vi "MASTER_QCM_O2_IM6_4200.vi"() -> ()   [LabVIEW 2013]
doc: "This example demonstrates temperature control and monitoring.\n\nNote:\nBefore start this VI is it necessary:\n\n- preconfigure some specific parameters that are not supported by this driver (e.g. PV-I/O Type, Linearization type, Alarm Input Values... ) by Quick Codes, or by Eurotherm iTools or by instrument front panel controls\n- enter correct VISA Resource Descriptor, Device Address and Baud Rate into front-panel controls"
uses:
  <vilib>/Instr/_visa.llb/VISA Event Mechanism.ctl
  <vilib>/Instr/_visa.llb/Select Event Type.ctl
  <vilib>/DAQmx/read.llb/DAQmx Read (Analog DBL 1Chan 1Samp).vi
  <vilib>/Utility/file.llb/Write To Spreadsheet File (string).vi
  LabVIEW Drivers for DVS instruments/Zahner VIs/IM/ZRemote-Globals.vi
  <vilib>/DAQmx/miscellaneous.llb/DAQmx Fill In Error Info.vi
panel:
  in  "Tab Control":T1(tab)
  in  "Add comments to the data file here and click anywhere outside the comment\nbox to save. The time at which the comment is saved is recorded in the data file.":string
  in  "O2 PUMP":bool
  in  "QCM":bool
  out "Program Errors":errorcluster
  out "Current Date/Time":string
  out "Starting Date/Time":string
  in  "Zahner IM6":bool
  in  "stop":bool
  in  "Quit VI":bool
  in  "Keithley 4200":bool
  out "Freq and Resistance Graph 2":T2(graph)
  out "Frequency (Hz)":dbl format="%.6e"
  out "Resistance (Ohm)":dbl format="%.6e"
  out "Waveform Chart 2":dbl(graph)
  out "Waveform Chart":cluster{dbl}(graph)
  out "Torr":dbl
  out "%":dbl
  out "atm":dbl
  out "O2 pump voltage":dbl format="%0.2f"
  in  "Com Port":i32(ring) items=["Com 1", "Com 2", "Com 3", "Com 4", "Com 5", "Com 6", "COM 7", "COM 8", "COM 9", "COM 10", "COM 11", "COM 12", "com 13", "COM 14"]
  in  "Baud Rate 2":i32(ring)=2 items=["2400", "4800", "9600", "19200", "38400", "57600", "115200"]
  out "Waveform Chart 3":cluster{dbl}(graph)
  out "XY Graph":cluster{dbl[], dbl[]}(graph)
  out "Current (A)    Voltage (V)":dbl[][](array[numeric]) caption="appended array"
  out "Resistance (Ohm)":dbl
  in  "Amplitude":dbl format="%.2p"
  in  "Period Count":i16=2 min=1 max=99
  in  "Frequency":dbl=1000.0 format="%.3p"
  out "Imaginary":dbl format="%.3p"
  out "Real":dbl format="%.3p"
  out "Potential Meter":dbl[unit](knob) scale=-10.0..10.0 scale format="%.0p"
  out "Current Meter":dbl[unit](knob) min=-2.0 max=2.0 step=1e-06 scale=-1e-06..1e-06 scale format="%.0p"
  in  "Measure OCP":bool
  in  "IP Address":string="127.0.0.1"
  in  "Device Name":string="ScriptRemote"
  in  "Galvanostat":bool
  in  "Set Current":dbl format="%.3p"
  in  "Potentiostat":bool=TRUE
  in  "Start IM remote":bool
  in  "Set Potential":dbl format="%.3p"
  in  "Device":i16 min=0 max=4
  in  "Measure EIS":bool
  in  "Cell Switch":bool
  in  "CV":bool
  in  "IE":bool
  in  "EIS":bool
  out "Busy":bool
  # "Configuring Instrument\n \nPlease Wait......\n\nChart will update in 20 sec"
  # "Instruments Connected"
  # "COMMENT BOX"
  # "Instructions:\n\nSelect the instruments above which are connected, turned on, and configured to record data.\n\nSet the file path destination for the data file produced by each instrument.\n\nRun the Pirani Control software, and make sure Pirani is saving a log of the temp/pressure/gas flow data. \n\nClick the RUN arrow on the LabVIEW toolbar, and wait for instruments to begin recording.\n\nTo end, click the red STOP button ONLY for instruments that are running.\n\nDO NOT press the STOP button on the toolbar."
  # "O2 Partial Pressure"
  # "V"
  # "4-Point Resistance Measurement:\nSMU1 = Current Source, Voltmeter\nSMU2 = COM & GND"
  # "Start Measurements"
  # "Impedance"
  # "Setup"
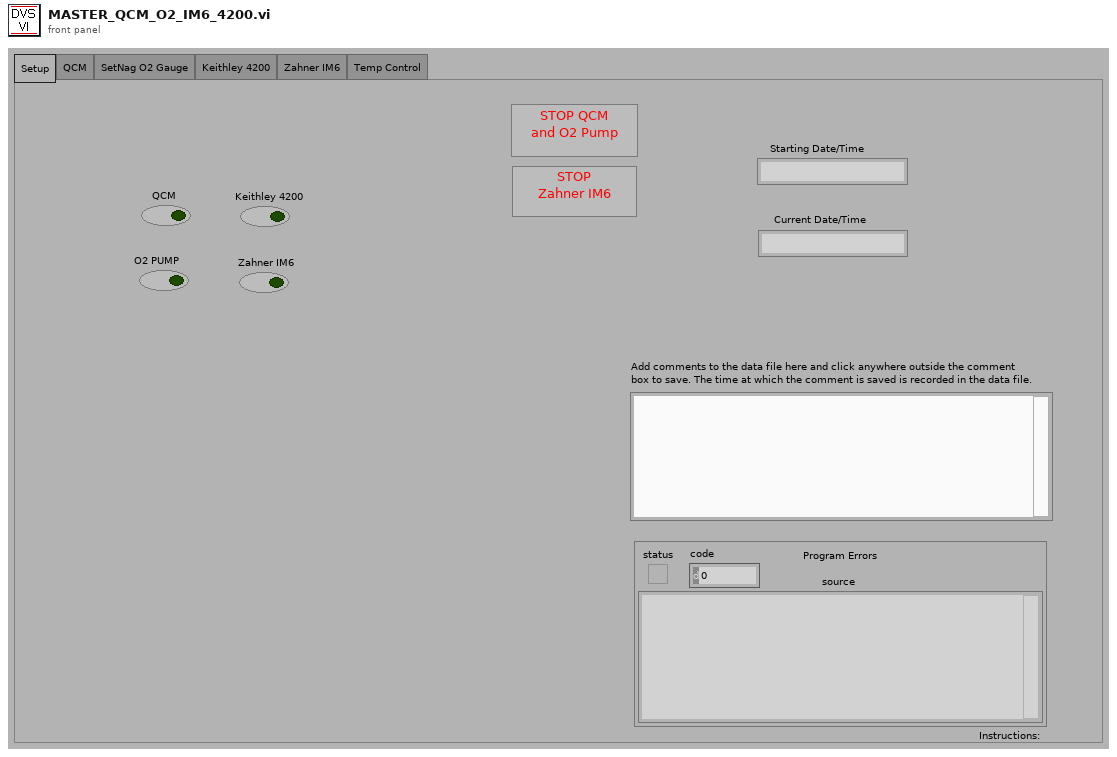
[diagram p1: front panel]
types:
  T1 = enum32{"Setup", "QCM", "SetNag O2 Gauge", "Keithley 4200", "Zahner IM6", "Temp Control"}
  T2 = cluster{"XY chart data":cluster{"x":dbl, "y":dbl}[]}[]
  T3 = enum16{"open", "open or create", "create or replace", "create", "open (read only)"}
  T4 = cluster{"IP Address":string, "Device Name":string, "Buffer Size":u16, "Start IM remote":bool}
  T5 = cluster{"Pset":dbl, "Cset":dbl, "Frq":dbl, "Ampl":dbl, "Nw":i16, "Pot":bool, "Gal":bool, "GAL":i16, "Cmin":dbl, "Cmax":dbl, "Pmin":dbl, "Pmax":dbl, "DEV":i16, "EPC":i16, "MAXDEV":i16}
  T6 = enum16{"no parity", "odd parity", "even parity", "mark parity", "space parity"}
  T7 = cluster{"Time Target (s)":dbl, "VISA in":refnum<visa-resource-name>, "error out":errorcluster}
  T8 = cluster{"Elapsed Time (s)":dbl, "VISA out":refnum<visa-resource-name>, "error out":errorcluster}
  T9 = typedef "Select Event Type.ctl" = u32
  T10 = typedef "VISA Event Mechanism.ctl" = u16
  T11 = cluster{"y":dbl, string, string, "error out":errorcluster}
  T12 = cluster{dbl, string, string, "error out":errorcluster}
  T13 = cluster{"error out":errorcluster, string, string}
  T14 = cluster{"timestamp out":dbl, "Frequency out":dbl}
  T15 = cluster{"timestamp out":dbl, "Resistance out":dbl}
  T16 = cluster{"error out":errorcluster, "error out":errorcluster, "error out":errorcluster}
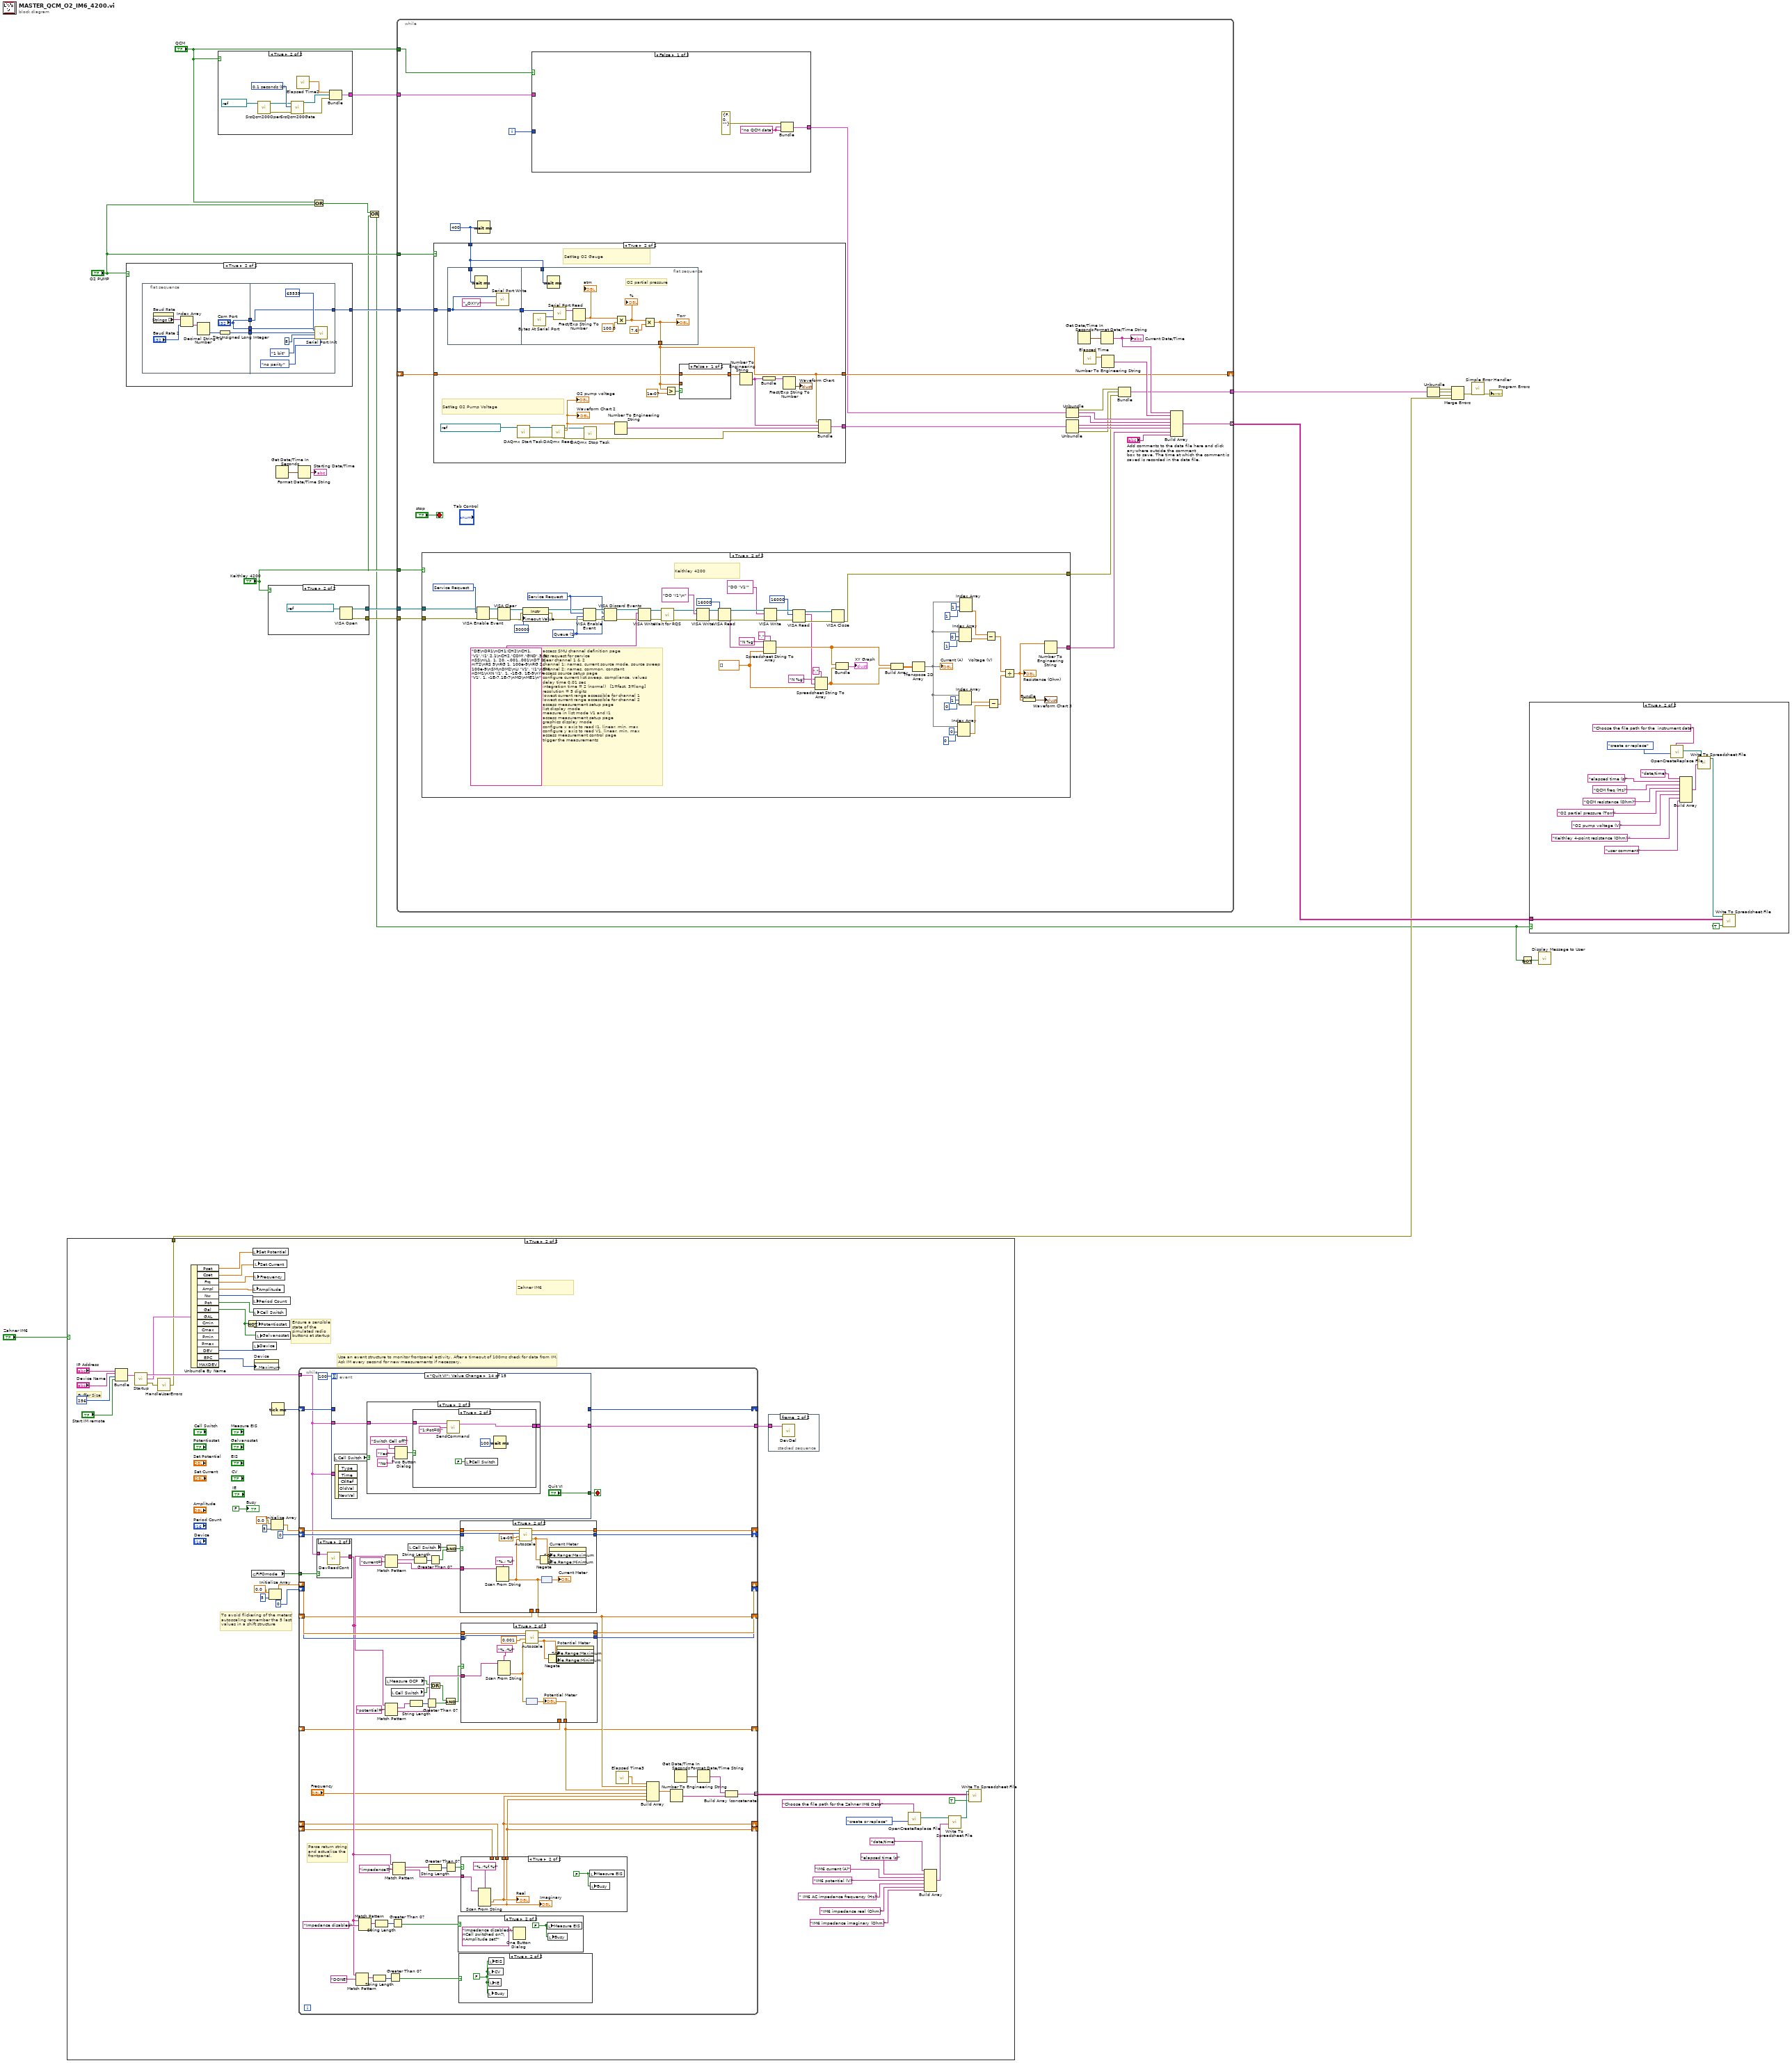
[diagram p0: block diagram]
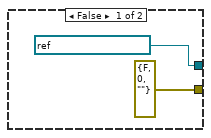
[diagram p2: hidden frame]
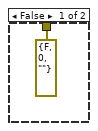
[diagram p4: hidden frame]
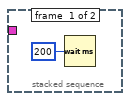
[diagram p5: hidden frame]
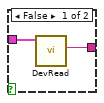
[diagram p7: hidden frame]
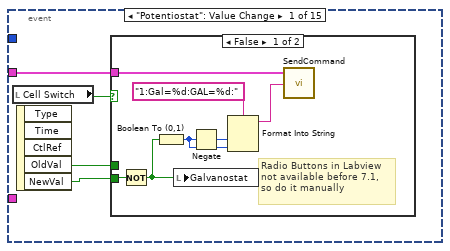
[diagram p12: hidden frame]
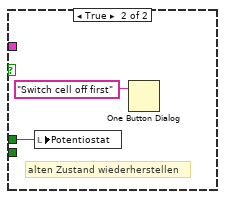
[diagram p13: hidden frame]
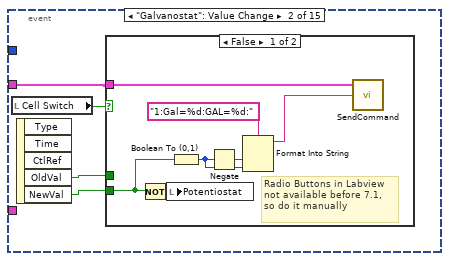
[diagram p14: hidden frame]
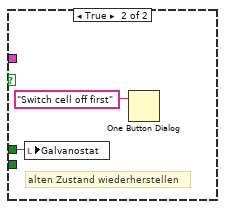
[diagram p15: hidden frame]
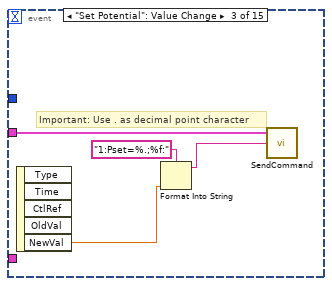
[diagram p16: hidden frame]
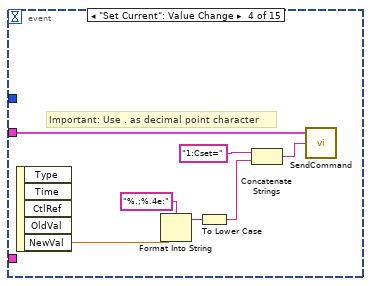
[diagram p17: hidden frame]
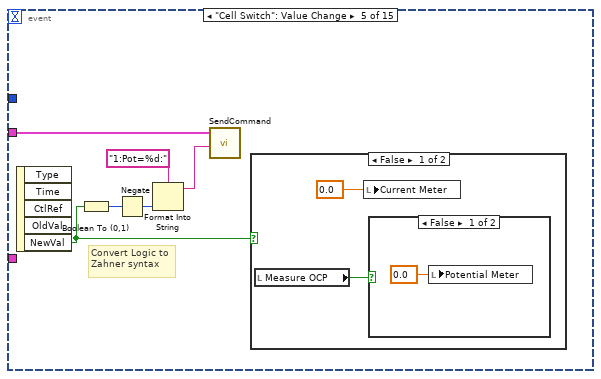
[diagram p18: hidden frame]
diagram:
  n1 = case shown="True" "Zahner IM6" {
    tunnel: [errorcluster {"status"=FALSE, "code"=0, "source"=""} ("error out") w23] -> w6
    frame False {
    }
    frame True {
      # "Zahner IM6"
      # "Use an event structure to monitor frontpanel activity. After a timeout of 100ms check for data from IM.\nAsk IM every second for new measurements if necessary."
      # "To avoid flickering of the meters'\nautoscaling remember the 5 last\nvalues in a shift structure"
      # "Buffer Size"
      # "Ensure a sensible\nstate of the\nsimulated radio\nbuttons at startup"
      n2 = Bundle("IP Address"="IP Address", "Device Name"="Device Name", "Buffer Size"=u16 256, "Start IM remote"="Start IM remote") -> (w62:T4)  [unwired: 1 in]
      n3 = call "Startup.vi"("Setup"=w62) -> ("error out"=w67:errorcluster, "ECWState"=w44:T5, "DevRefOut"=w61:cluster{"DevIdxOut":u8, "ReadBuffer":string})  [unwired: 2 in]
      n4 = call "HandleUserErrors.vi"("error in (no error)"=w67) -> ("error out"=w23:errorcluster)
      n5 = Unbundle By Name(w44) -> ("Pset"=w50:dbl, "Cset"=w49:dbl, "Frq"=w48:dbl, "Ampl"=w47:dbl, "Nw"=w46:i16, "Pot"=w43:bool, "Gal"=w41:bool, "DEV"=w45:i16, "MAXDEV"=w39:i16)  [unwired: 6 out]
      n6 = Not(x=w41) -> (.not. x?=w42:bool)
      n7 = global read "ZRemote-Globals.vi" "FIFOmode"() -> (w40:bool)
      n8 = local write "Set Potential"(w50) -> ()
      n9 = local write "Amplitude"(w47) -> ()
      n10 = local write "Period Count"(w46) -> ()
      n11 = local write "Device"(w45) -> ()
      n12 = local write "Frequency"(w48) -> ()
      n13 = local write "Cell Switch"(w43) -> ()
      n14 = local write "Set Current"(w49) -> ()
      n15 = property on="Device" class="DigNum (strict)"("Data Entry Limits:Maximum"=w39) -> ()  [unwired: 2 in, 2 out]
      n16 = local write "Potentiostat"(w42) -> ()
      n17 = local write "Galvanostat"(w41) -> ()
      n18 = Initialize Array(0.0 ("element"), 5 ("dimension size")) -> (w53:dbl[])
      n19 = Initialize Array(0.0 ("element"), 5 ("dimension size")) -> (w57:dbl[])
      n20 = Tick Count (ms)() -> (millisecond timer value=w52:u32)
      n21 = while {
        tunnel: w61 -> [w99]
        shift-right: [w110] -> _
        shift-left: u32 0 -> [w111]
        shift-right: [w108] -> _
        shift-left: w57 -> [w109]
        shift-right: [w107] -> _
        shift-left: w53 -> [w105]
        shift-right: [w106] -> _
        shift-left: u32 0 -> [w104]
        shift-right: [w101] -> _
        shift-left: w52 -> [w102]
        tunnel: [w100] -> w51
        tunnel: w40 -> [w98]
        shift-right: [w76] -> _
        shift-left: _ -> [w84]
        shift-right: [w75] -> _
        shift-left: _ -> [w83]
        shift-right: [w82] -> _
        shift-left: _ -> [w81]
        shift-right: [w80] -> _
        shift-left: _ -> [w79]
        tunnel: [w70] -> w31 mode=indexing
        stop <- w129 stop-if-true
        # "Parse return string\nand actualize the\nfrontpanel."
        n22 = case shown="True" w98 {
          tunnel: w99 -> [w132 w134]
          tunnel: [w131 w133] -> w86
          frame False {
            n23 = call "DevRead.vi"("DevRefIn"=w132) -> ("Data"=w131:string)  [unwired: 4 in, 2 out]
          }
          frame True {
            n24 = call "DevReadCont.vi"("DevRefIn"=w134) -> ("Data"=w133:string)  [unwired: 4 in, 2 out]
          }
        }
        n25 = event shown="[13] \"Quit VI\": Value Change" {
          selector: _ -> [_ _ _ _ _ _ _ _ _ _ _ _ _ _ _]
          dyn-events: _ -> [_ _ _ _ _ _ _ _ _ _ _ _ _ _ _]
          timeout: 100 -> [_ _ _ _ _ _ _ _ _ _ _ _ _ _ _]
          tunnel: [_ _ _ _ _ _ _ _ _ _ _ _ _ "Quit VI" _] -> w129
          tunnel: w99 -> [w172 w185 w201 w208 w212 w220 w223 w226 w229 w236 w242 w246 _ w285 w307]
          tunnel: w99 -> [_ _ _ _ _ _ _ _ _ _ _ _ w250 _ w306]
          tunnel: w102 -> [_ _ _ _ _ _ _ _ _ _ _ _ _ _ w304]
          tunnel: [_ _ _ _ _ _ _ _ _ _ _ _ _ _ w305] -> w101
          tunnel: [_ _ _ _ _ _ _ _ _ _ _ _ _ w283 _] -> w100
          event "Potentiostat": Value Change {
            n26 = local read "Cell Switch"() -> (w175:bool)
            n27 = event-data() -> ("OldVal"=w173:bool, "NewVal"=w174:bool)  [unwired: 1 in, 3 out]
            n28 = case shown="False" w175 {
              tunnel: w174 -> [w180 _]
              tunnel: w173 -> [_ w183]
              tunnel: w172 -> [w182 _]
              frame False {
                # "Radio Buttons in Labview\nnot available before 7.1,\nso do it manually"
                n29 = Not(x=w180) -> (.not. x?=w179:bool)
                n30 = Boolean To (0,1)(Boolean=w179) -> (0, 1=w176:i16)
                n31 = local write "Galvanostat"(w179) -> ()
                n32 = Negate(x=w176) -> (-x=w177:i16)
                n33 = Format Into String(format string="1:Gal=%d:GAL=%d:", w177, w176) -> (resulting string=w178:string)  [unwired: 2 in, 1 out]
                n34 = call "SendCommand.vi"("Command"=w178, "DevRefIn"=w182) -> ()  [unwired: 1 in, 2 out]
              }
              frame True {
                # "alten Zustand wiederherstellen"
                n35 = local write "Potentiostat"(w183) -> ()
                n36 = One Button Dialog(message="Switch cell off first") -> ()  [unwired: 1 in, 1 out]
              }
            }
          }
          event "Galvanostat": Value Change {
            n37 = local read "Cell Switch"() -> (w188:bool)
            n38 = event-data() -> ("OldVal"=w186:bool, "NewVal"=w187:bool)  [unwired: 1 in, 3 out]
            n39 = case shown="False" w188 {
              tunnel: w187 -> [w192 _]
              tunnel: w186 -> [_ w196]
              tunnel: w185 -> [w191 _]
              frame False {
                # "Radio Buttons in Labview\nnot available before 7.1,\nso do it manually"
                n40 = Not(x=w192) -> (.not. x?=w193:bool)
                n41 = local write "Potentiostat"(w193) -> ()
                n42 = Boolean To (0,1)(Boolean=w192) -> (0, 1=w189:i16)
                n43 = Negate(x=w189) -> (-x=w190:i16)
                n44 = Format Into String(format string="1:Gal=%d:GAL=%d:", w190, w189) -> (resulting string=w194:string)  [unwired: 2 in, 1 out]
                n45 = call "SendCommand.vi"("Command"=w194, "DevRefIn"=w191) -> ()  [unwired: 1 in, 2 out]
              }
              frame True {
                # "alten Zustand wiederherstellen"
                n46 = local write "Galvanostat"(w196) -> ()
                n47 = One Button Dialog(message="Switch cell off first") -> ()  [unwired: 1 in, 1 out]
              }
            }
          }
          event "Set Potential": Value Change {
            # "Important: Use . as decimal point character"
            n48 = event-data() -> ("NewVal"=w198:dbl)  [unwired: 1 in, 4 out]
            n49 = Format Into String(format string="1:Pset=%.;%f:", w198) -> (resulting string=w199:string)  [unwired: 2 in, 1 out]
            n50 = call "SendCommand.vi"("Command"=w199, "DevRefIn"=w201) -> ()  [unwired: 1 in, 2 out]
          }
          event "Set Current": Value Change {
            # "Important: Use . as decimal point character"
            n51 = event-data() -> ("NewVal"=w206:dbl)  [unwired: 1 in, 4 out]
            n52 = Format Into String(format string="%.;%.4e:", w206) -> (resulting string=w203:string)  [unwired: 2 in, 1 out]
            n53 = To Lower Case(string=w203) -> (all lower case string=w202:string)
            n54 = Concatenate Strings("1:Cset=" ("format string"), w202) -> (w205:string)
            n55 = call "SendCommand.vi"("Command"=w205, "DevRefIn"=w208) -> ()  [unwired: 1 in, 2 out]
          }
          event "Cell Switch": Value Change {
            # "Convert Logic to Zahner syntax"
            n56 = event-data() -> ("NewVal"=w211:bool)  [unwired: 1 in, 4 out]
            n57 = Boolean To (0,1)(Boolean=w211) -> (0, 1=w209:i16)
            n58 = Negate(x=w209) -> (-x=w210:i16)
            n59 = Format Into String(format string="1:Pot=%d:", w210) -> (resulting string=w214:string)  [unwired: 2 in, 1 out]
            n60 = call "SendCommand.vi"("Command"=w214, "DevRefIn"=w212) -> ()  [unwired: 1 in, 2 out]
            n61 = case shown="False" w211 {
              frame False {
                n62 = local read "Measure OCP"() -> (w215:bool)
                n63 = local write "Current Meter"(dbl[unit] 0.0 ("Current Meter")) -> ()
                n64 = case shown="False" w215 {
                  frame False {
                    n65 = local write "Potential Meter"(dbl[unit] 0.0 ("Potential Meter")) -> ()
                  }
                  frame True {
                  }
                }
              }
              frame True {
              }
            }
          }
          event "Measure EIS": Value Change {
            n66 = event-data() -> ()  [unwired: 1 in, 5 out]
            n67 = call "SendCommand.vi"("Command"="1:IMPEDANCE:" ("format string"), "DevRefIn"=w220) -> ()  [unwired: 1 in, 2 out]
            n68 = local write "Busy"(TRUE ("Busy")) -> ()
          }
          event "EIS": Value Change {
            n69 = event-data() -> ()  [unwired: 1 in, 5 out]
            n70 = call "SendCommand.vi"("Command"="1:EIS:" ("format string"), "DevRefIn"=w223) -> ()  [unwired: 1 in, 2 out]
            n71 = local write "Busy"(TRUE ("Busy")) -> ()
          }
          event "IE": Value Change {
            n72 = event-data() -> ()  [unwired: 1 in, 5 out]
            n73 = call "SendCommand.vi"("Command"="1:IE:" ("format string"), "DevRefIn"=w226) -> ()  [unwired: 1 in, 2 out]
            n74 = local write "Busy"(TRUE ("Busy")) -> ()
          }
          event "CV": Value Change {
            n75 = event-data() -> ()  [unwired: 1 in, 5 out]
            n76 = call "SendCommand.vi"("Command"="1:CV:" ("format string"), "DevRefIn"=w229) -> ()  [unwired: 1 in, 2 out]
            n77 = local write "Busy"(TRUE ("Busy")) -> ()
          }
          event "Frequency": Value Change {
            # "Important: Use . as decimal point character"
            n78 = event-data() -> ("NewVal"=w230:dbl)  [unwired: 1 in, 4 out]
            n79 = Format Into String(format string="%.;%e:", w230) -> (resulting string=w233:string)  [unwired: 2 in, 1 out]
            n80 = To Lower Case(string=w233) -> (all lower case string=w232:string)
            n81 = Concatenate Strings("1:Frq=" ("format string"), w232) -> (w231:string)
            n82 = call "SendCommand.vi"("Command"=w231, "DevRefIn"=w236) -> ()  [unwired: 1 in, 2 out]
          }
          event "Amplitude": Value Change {
            # "convert V to mV"
            # "Important: Use . as decimal point character"
            n83 = event-data() -> ("NewVal"=w239:dbl)  [unwired: 1 in, 4 out]
            n84 = Multiply(x=w239, y=1000.0) -> (x*y=w238:dbl)
            n85 = Format Into String(format string="1:Ampl=%.;%f:", w238) -> (resulting string=w240:string)  [unwired: 2 in, 1 out]
            n86 = call "SendCommand.vi"("Command"=w240, "DevRefIn"=w242) -> ()  [unwired: 1 in, 2 out]
          }
          event "Period Count": Value Change {
            # "Important: Use . as decimal point character"
            n87 = event-data() -> ("NewVal"=w243:i16)  [unwired: 1 in, 4 out]
            n88 = Format Into String(format string="1:Nw=%.;%d:", w243) -> (resulting string=w244:string)  [unwired: 2 in, 1 out]
            n89 = call "SendCommand.vi"("Command"=w244, "DevRefIn"=w246) -> ()  [unwired: 1 in, 2 out]
          }
          event "Device": Value Change {
            n90 = event-data() -> ("NewVal"=w265:i16)  [unwired: 1 in]
            n91 = Format Into String(format string="1:DEV%%=%d:", w265) -> (resulting string=w266:string)  [unwired: 2 in, 1 out]
            n92 = call "SendCommand.vi"("GetACK"=TRUE, "Command"=w266, "DevRefIn"=w250) -> ("Result"=w249:string, "DevRefOut"=w248:cluster{"DevIdxOut":u8, "ReadBuffer":string})
            n93 = case shown="\"device not present\"" w249 {
              tunnel: w248 -> [w268 w271 w282]
              tunnel: [w268 w270 w282] -> w247
              frame "device not present" {
                n94 = One Button Dialog(message="Error: Cannot change device!") -> ()  [unwired: 1 in, 1 out]
              }
              frame "", Default {
                n95 = while {
                  tunnel: w271 -> [w277]
                  tunnel: [w275] -> w270
                  i -> [w272]
                  stop <- w278 continue-if-true
                  # "Wait max. 30s until\nEPC device has booted."
                  n96 = Wait (ms)(milliseconds to wait=u32 10) -> ()  [unwired: 1 out]
                  n97 = call "DevReadCont.vi"("DevRefIn"=w277) -> ("Data"=w280:string, "DevRefOut"=w275:cluster{"DevIdxOut":u8, "ReadBuffer":string})  [unwired: 4 in, 1 out]
                  n98 = String Length(string=w280) -> (length=w279:i32)
                  n99 = Less?(x=w272, y=3000) -> (x < y?=w273:bool)
                  n100 = Equal To 0?(x=w279) -> (x = 0?=w274:bool)
                  n101 = And(x=w273, y=w274) -> (x .and. y?=w278:bool)
                }
              }
              frame "ok" {
              }
            }
            n102 = call "SendCommand.vi"("GetACK"=TRUE, "Command"="1:SENDSETUP:", "DevRefIn"=w247) -> ("Result"=w251:string)  [unwired: 1 out]
            n103 = call "GetECWState.vi"("String"=w251) -> ("ECWState"=w261:T5)
            n104 = Unbundle By Name(w261) -> ("Pset"=w260:dbl, "Cset"=w259:dbl, "Frq"=w258:dbl, "Ampl"=w257:dbl, "Nw"=w256:i16, "Pot"=w255:bool, "Gal"=w253:bool, "DEV"=w252:i16)
            n105 = Not(x=w253) -> (.not. x?=w254:bool)
            n106 = local write "Amplitude"(w257) -> ()
            n107 = local write "Period Count"(w256) -> ()
            n108 = local write "Cell Switch"(w255) -> ()
            n109 = local write "Set Potential"(w260) -> ()
            n110 = local write "Frequency"(w258) -> ()
            n111 = local write "Galvanostat"(w253) -> ()
            n112 = local write "Set Current"(w259) -> ()
            n113 = local write "Device"(w252) -> ()
            n114 = local write "Potentiostat"(w254) -> ()
          }
          event "Quit VI": Value Change {
            n115 = local read "Cell Switch"() -> (w286:bool)
            n116 = event-data() -> ()  [unwired: 1 in, 5 out]
            n117 = case shown="True" w286 {
              tunnel: w285 -> [w287 w289]
              tunnel: [w287 w288] -> w283
              frame False {
              }
              frame True {
                n118 = Two Button Dialog(message="Switch Cell off?", 1:"No" ("F button name (\"Cancel\")"), 2:"Yes" ("T button name (\"OK\")")) -> (T button?=w290:bool)
                n119 = case shown="True" w290 {
                  tunnel: w289 -> [w294 w299]
                  tunnel: [w294 w296] -> w288
                  frame False {
                  }
                  frame True {
                    n120 = call "SendCommand.vi"("Command"="1:Pot=0:" ("Data"), "DevRefIn"=w299) -> ("DevRefOut"=w296:cluster{"DevIdxOut":u8, "ReadBuffer":string})  [unwired: 1 in, 1 out]
                    n121 = local write "Cell Switch"(FALSE ("Cell Switch")) -> ()
                    n122 = Wait (ms)(milliseconds to wait=u32 100) -> ()  [unwired: 1 out]
                  }
                }
              }
            }
          }
          event Timeout {
            n123 = event-data() -> ("Time"=w300:u32)  [unwired: 1 in]
            n124 = Subtract(x=w300, y=w304) -> (x-y=w303:u32)
            n125 = Greater Or Equal?(x=w303, y=u32 1000) -> (x >= y?=w301:bool)
            n126 = case shown="True" w301 {
              tunnel: w307 -> [_ w312]
              tunnel: w306 -> [_ w311]
              tunnel: w304 -> [w308 _]
              tunnel: [w308 w310] -> w305
              tunnel: w300 -> [_ w310]
              frame False {
              }
              frame True {
                n127 = local read "Busy"() -> (w309:bool)
                n128 = local read "Cell Switch"() -> (w315:bool)
                n129 = local read "Cell Switch"() -> (w316:bool)
                n130 = Not(x=w309) -> (.not. x?=w317:bool)
                n131 = Not(x=w315) -> (.not. x?=w314:bool)
                n132 = And(x=w316, y=w317) -> (x .and. y?=w318:bool)
                n133 = And(x="Measure OCP", y=w314) -> (x .and. y?=w319:bool)
                n134 = case shown="True" w318 {
                  tunnel: w312 -> [_ w321]
                  frame False {
                  }
                  frame True {
                    n135 = call "SendCommand.vi"("GetACK"=FALSE, "Command"="1:CURRENT:POTENTIAL:" ("format string"), "DevRefIn"=w321) -> ()  [unwired: 2 out]
                  }
                }
                n136 = case shown="True" w319 {
                  tunnel: w311 -> [_ w324]
                  frame False {
                  }
                  frame True {
                    n137 = call "SendCommand.vi"("GetACK"=FALSE, "Command"="1:POTENTIAL:" ("format string"), "DevRefIn"=w324) -> ()  [unwired: 2 out]
                  }
                }
              }
            }
          }
        }
        n138 = Match Pattern(string=w86, regular expression="DONE") -> (match substring=w89:string)  [unwired: 1 in, 3 out]
        n139 = Match Pattern(string=w86, regular expression="Impedance disabled") -> (match substring=w115:string)  [unwired: 1 in, 3 out]
        n140 = String Length(string=w89) -> (length=w88:i32)
        n141 = String Length(string=w115) -> (length=w114:i32)
        n142 = Match Pattern(string=w86, regular expression="current=") -> (match substring=w126:string, after substring=w124:string)  [unwired: 1 in, 2 out]
        n143 = Match Pattern(string=w86, regular expression="potential=") -> (match substring=w123:string, after substring=w121:string)  [unwired: 1 in, 2 out]
        n144 = local read "Measure OCP"() -> (w92:bool)
        n145 = Greater Than 0?(x=w88) -> (x > 0?=w85:bool)
        n146 = local read "Cell Switch"() -> (w91:bool)
        n147 = Greater Than 0?(x=w114) -> (x > 0?=w112:bool)
        n148 = Match Pattern(string=w86, regular expression="impedance=") -> (match substring=w120:string, after substring=w116:string)  [unwired: 1 in, 2 out]
        n149 = local read "Cell Switch"() -> (w95:bool)
        n150 = String Length(string=w123) -> (length=w103:i32)
        n151 = String Length(string=w126) -> (length=w125:i32)
        n152 = Greater Than 0?(x=w103) -> (x > 0?=w93:bool)
        n153 = Greater Than 0?(x=w125) -> (x > 0?=w96:bool)
        n154 = String Length(string=w120) -> (length=w119:i32)
        n155 = Or(x=w92, y=w91) -> (x .or. y?=w90:bool)
        n156 = And(x=w90, y=w93) -> (x .and. y?=w94:bool)
        n157 = Greater Than 0?(x=w119) -> (x > 0?=w117:bool)
        n158 = And(x=w95, y=w96) -> (x .and. y?=w97:bool)
        n159 = case shown="True" w112 {
          frame False {
          }
          frame True {
            w135 = FALSE ("Measure EIS")
            n160 = One Button Dialog(message="Impedance disabled!\nCell switched on?\nAmplitude set?") -> ()  [unwired: 1 in, 1 out]
            n161 = local write "Measure EIS"(w135) -> ()
            n162 = local write "Busy"(w135) -> ()
          }
        }
        n163 = case shown="True" w85 {
          frame False {
          }
          frame True {
            w130 = FALSE ("EIS")
            n164 = local write "CV"(w130) -> ()
            n165 = local write "Busy"(w130) -> ()
            n166 = local write "EIS"(w130) -> ()
            n167 = local write "IE"(w130) -> ()
          }
        }
        n168 = case shown="True" w97 {
          tunnel: w124 -> [_ w170]
          tunnel: w111 -> [w160 w163]
          tunnel: [w160 w164] -> w110
          tunnel: w109 -> [w159 w168]
          tunnel: [w159 w167] -> w108
          tunnel: [w158 w161] -> w82
          tunnel: w81 -> [w158 _]
          frame False {
          }
          frame True {
            n169 = Scan From String(format string="%.; %f", input string=w170) -> (output 1=w161:dbl)  [unwired: 3 in, 3 out]
            n170 = call "Autoscale.vi"("New Value"=w161, "Min Scale"=1e-09, "Old Position"=w163, "Input Ringbuffer"=w168) -> ("Maximum"=w165:dbl, "New Position"=w164:u32, "Output Ringbuffer"=w167:dbl[])
            n171 = Negate(x=w165) -> (-x=w166:dbl)
            n172 = node(w161) -> (→"Current Meter":dbl[unit])
            n173 = property on="Current Meter" class="Knob (strict)"("Scale.Range:Maximum"=w165, "Scale.Range:Minimum"=w166) -> ()  [unwired: 2 in, 2 out]
          }
        }
        n174 = case shown="True" w117 {
          tunnel: w116 -> [_ w142]
          tunnel: [w137 w140] -> w75
          tunnel: [w138 w139] -> w76
          tunnel: w84 -> [w138 _]
          tunnel: w83 -> [w137 _]
          frame False {
            # "Switch EIS Mode off again"
          }
          frame True {
            w141 = FALSE ("Measure EIS")
            n175 = Scan From String(format string="%.;%f,%f", input string=w142) -> (output 1=w140:dbl, output 2=w139:dbl)  [unwired: 4 in, 3 out]
            "Real" <- w140
            "Imaginary" <- w139
            n176 = local write "Measure EIS"(w141) -> ()
            n177 = local write "Busy"(w141) -> ()
          }
        }
        n178 = case shown="True" w94 {
          tunnel: w121 -> [_ w156]
          tunnel: [w146 w150] -> w107
          tunnel: [w145 w151] -> w106
          tunnel: w105 -> [w146 w154]
          tunnel: w104 -> [w145 w149]
          tunnel: [w144 w147] -> w80
          tunnel: w79 -> [w144 _]
          frame False {
          }
          frame True {
            n179 = Scan From String(format string="%.;%f", input string=w156) -> (output 1=w147:dbl)  [unwired: 3 in, 3 out]
            n180 = call "Autoscale.vi"("New Value"=w147, "Min Scale"=0.001, "Old Position"=w149, "Input Ringbuffer"=w154) -> ("Maximum"=w152:dbl, "New Position"=w151:u32, "Output Ringbuffer"=w150:dbl[])
            n181 = node(w147) -> (→"Potential Meter":dbl[unit])
            n182 = Negate(x=w152) -> (-x=w153:dbl)
            n183 = property on="Potential Meter" class="Knob (strict)"("Scale.Range:Maximum"=w152, "Scale.Range:Minimum"=w153) -> ()  [unwired: 2 in, 2 out]
          }
        }
        n184 = call "Elapsed Time3"() -> ("Elapsed Time (s)"=w77:dbl)  [unwired: 12 in, 7 out]
        n185 = Build Array(w77, w82, w80, "Frequency", w75, w76) -> (w78:dbl[])
        n186 = Number To Engineering String(4:w78) -> (0:w72:string[])  [unwired: 3 in]
        n187 = Get Date/Time In Seconds() -> (seconds since 1Jan1904=w73:timestamp)
        n188 = Format Date/Time String(seconds (now)=w73) -> (date/time string=w71:string)  [unwired: 2 in]
        n189 = Build Array (concatenate)(w71, w72) -> (w70:string[])
      }
      n190 = stacked-sequence {
        tunnel: w51 -> [_ w69]
        frame #0 {
          n191 = Wait (ms)(milliseconds to wait=u32 200) -> ()  [unwired: 1 out]
        }
        frame #1 {
          n192 = call "DevDel.vi"("DevRefIn"=w69) -> ()  [unwired: 6 in, 1 out]
        }
      }
      n193 = call <instrlib>:"OpenCreateReplace File.vi"("prompt"="Choose the file path for the Zahner IM6 Data", "function (open:0)"=T3."create or replace") -> ("new file path"=w25:path)  [unwired: 6 in, 3 out]
      n194 = Build Array("date/time", "elapsed time (s)", "IM6 current (A)", "IM6 potential (V)", " IM6 AC impedance frequency (Hz)" ("element"), "IM6 impedance real (Ohm)" ("element"), "IM6 impedance imaginary (Ohm)" ("element")) -> (w37:string[])
      n195 = call-poly <vilib>:"Write To Spreadsheet File.vi"("1D data"=w37, "file path (dialog if empty)"=w25) -> ("new file path (Not A Path if cancelled)"=w36:path)  [unwired: 6 in]
      n196 = call-poly <vilib>:"Write To Spreadsheet File.vi"("append to file? (new file:F)"=TRUE, "2D data"=w31, "file path (dialog if empty)"=w36) -> ()  [unwired: 5 in, 1 out]
      "Busy" <- FALSE ("Busy")
    }
  }
  n197 = case shown="True" "O2 PUMP" {
    tunnel: [w326 w327] -> w18
    frame False {
      w326 = 0 items=["Com 1", "Com 2", "Com 3", "Com 4", "Com 5", "Com 6", "COM 7", "COM 8", "COM 9", "COM 10", "COM 11", "COM 12", "com 13", "COM 14"] ("Com Port 3")
    }
    frame True {
      n198 = flat-sequence {
        tunnel: ["Com Port"] -> w330
        tunnel: [w332] -> w329
        tunnel: ["Com Port"] -> w328
        tunnel: w330 -> [w339]
        tunnel: w329 -> [w338]
        tunnel: w328 -> [w337]
        tunnel: [w337] -> w327
        frame #0 {
          n199 = property on="Baud Rate" class="Ring (strict)"() -> ("Strings []"=w334:string[])  [unwired: 2 in, 2 out]
          n200 = Index Array(array=w334, index="Baud Rate 2") -> (element=w335:string)
          n201 = Decimal String To Number(string=w335) -> (number=w333:i32)  [unwired: 2 in, 1 out]
          n202 = To Unsigned Long Integer(number=w333) -> (unsigned 32bit integer=w332:u32)
        }
        frame #1 {
          n203 = call <vilib>:"Serial Port Init.vi"("parity"=T6."no parity", "buffer size"=u16 65535, "stop bits"=enum16{"1 bit", "1.5 bits", "2 bits"}."1 bit", "data bits"=u16 8, "baud rate"=w338, "port number"=w339) -> ()  [unwired: 1 in, 1 out]
        }
      }
    }
  }
  n204 = case shown="True" "QCM" {
    tunnel: [w344 w348] -> w17
    frame False {
      n205 = Bundle("Time Target (s)"=0.0, "VISA in"=refnum<visa-resource-name> "COM6", "error out"=errorcluster {"status"=FALSE, "code"=0, "source"=""}) -> (w344:T7)  [unwired: 1 in]
    }
    frame True {
      w355 = u16 0 items=["0.1 seconds", "1.0 seconds", "10.0 seconds"] ("Gate in")
      n206 = call <instrlib>:"SrsQcm200Open.vi"("VISA in"=refnum<visa-resource-name> "COM6") -> ("error out"=w352:errorcluster, "VISA out"=w353:refnum<visa-resource-name>)  [unwired: 4 in]
      n207 = call <instrlib>:"SrsQcm200Gate.vi"("VISA in"=w353, "Gate in"=w355, "error in (no error)"=w352) -> ("VISA out"=w350:refnum<visa-resource-name>, "error out"=w349:errorcluster)  [unwired: 14 in, 1 out]
      n208 = call "Elapsed Time2"() -> ("Elapsed Time (s)"=w351:dbl)  [unwired: 12 in, 7 out]
      n209 = Bundle("Elapsed Time (s)"=w351, "VISA out"=w350, "error out"=w349) -> (w348:T8)  [unwired: 1 in]
    }
  }
  n210 = case shown="True" "Keithley 4200" {
    tunnel: [refnum<visa-resource-name> "GPIB0::17::INSTR" ("VISA resource name") w359] -> w8
    tunnel: [errorcluster {"status"=FALSE, "code"=0, "source"=""} ("error out") w358] -> w7
    frame False {
    }
    frame True {
      n211 = VISA Open(VISA resource name=refnum<visa-resource-name> "GPIB0::17::INSTR") -> (VISA resource name=w359:refnum<visa-resource-name>, error out=w358:errorcluster)  [unwired: 1 in, 3 out]
    }
  }
  n212 = Get Date/Time In Seconds() -> (seconds since 1Jan1904=w20:timestamp)
  n213 = Format Date/Time String(seconds (now)=w20) -> (date/time string=→"Starting Date/Time":string)  [unwired: 2 in]
  n214 = Or(x="QCM", y="O2 PUMP") -> (x .or. y?=w5:bool)
  n215 = Or(x=w5, y="Keithley 4200") -> (x .or. y?=w3:bool)
  n216 = while {
    shift-right: [w385] -> _
    shift-left: _ -> [w384]
    tunnel: w18 -> [w379]
    tunnel: w17 -> [w374]
    tunnel: [w370] -> w16
    tunnel: [w367] -> w11 mode=indexing
    tunnel: "QCM" -> [w368]
    tunnel: "O2 PUMP" -> [w363]
    tunnel: w8 -> [w366]
    tunnel: w7 -> [w365]
    tunnel: "Keithley 4200" -> [w364]
    i -> [w383]
    stop <- "stop" stop-if-true
    w382 = u32 400 ("milliseconds to wait")
    n217 = case shown="True" w364 {
      tunnel: w366 -> [_ w397]
      tunnel: w365 -> [_ w396]
      tunnel: ["no Keithley 4200 data" w395] -> w362
      tunnel: [errorcluster {"status"=FALSE, "code"=0, "source"=""} ("error out") w394] -> w361
      frame False {
      }
      frame True {
        w407 = T9 1073684491 items=["Service Request"=1073684491, "Trigger"=3221168138, "Clear"=1073684493, "VXI Signal"=1073684512, "VXI/VME Interrupt"=3221168161, "VXI/VME Sysfail"=1073684509, "VXI/VME Sysreset"=1073684510, "GPIB CIC"=1073684498, "GPIB Talk"=1073684499, "GPIB Listen"=1073684500, "PXI Interrupt"=1073684514, "Serial Break"=1073684515, "Serial TermChar"=1073684516, "Serial CTS"=1073684521, "Serial DSR"=1073684522, "Serial DCD"=1073684524, "Serial RI"=1073684526, "Serial Character"=1073684533, "USB Interrupt"=1073684535, "All Enabled"=1073709055] ("Event Type")
        w414 = T10 1 items=["Queue"=1] ("Mechanism Type")
        w415 = T9 1073684491 items=["Service Request"=1073684491, "Trigger"=3221168138, "Clear"=1073684493, "VXI Signal"=1073684512, "VXI/VME Interrupt"=3221168161, "VXI/VME Sysfail"=1073684509, "VXI/VME Sysreset"=1073684510, "GPIB CIC"=1073684498, "GPIB Talk"=1073684499, "GPIB Listen"=1073684500, "PXI Interrupt"=1073684514, "Serial Break"=1073684515, "Serial TermChar"=1073684516, "Serial CTS"=1073684521, "Serial DSR"=1073684522, "Serial DCD"=1073684524, "Serial RI"=1073684526, "Serial Character"=1073684533, "USB Interrupt"=1073684535, "All Enabled"=1073709055] ("Event Type")
        w442 = dbl[] []
        # "Keithley 4200"
        # "access SMU channel definition page\nset request for service\nclear channel 1 & 2\nchannel 1: names, current source mode, source sweep\nchannel 2: names, common, constant\naccess source setup page\nconfigure current list sweep, compliance, values\ndelay time 0.01 sec\nintegration time = 2 (normal)   [1=fast, 3=long]\nresolution = 5 digits\nlowest current range accessible for channel 1\nlowest current range accessible for channel 2\naccess measurement setup page\nlist display mode\nmeasure in list mode V1 and I1\naccess measurement setup page\ngraphics display mode\nconfigure x axis to read I1, linear, min, max\nconfigure y axis to read V1, linear, min, max\naccess measurement control page\ntrigger the measurements"
        n218 = VISA Enable Event(8:w396, 10:w407, 11:w397) -> (0:w408:errorcluster, 3:w409:refnum<visa-resource-name>)  [unwired: 1 out]
        n219 = VISA Clear(VISA resource name=w409, error in (no error)=w408) -> (VISA resource name out=w413:refnum<visa-resource-name>, error out=w412:errorcluster)
        n220 = property class="Instr"(reference=w413, error in=w412, "General Settings:Timeout Value"=u32 30000) -> (reference out=w411:refnum<visa-resource-name>, error out=w410:errorcluster)
        n221 = VISA Enable Event(8:w410, 9:w414, 10:w415, 11:w411) -> (0:w416:errorcluster, 3:w417:refnum<visa-resource-name>)
        n222 = VISA Discard Events(8:w416, 9:w414, 10:w415, 11:w417) -> (0:w402:errorcluster, 3:w403:refnum<visa-resource-name>)
        n223 = VISA Write(VISA resource name=w403, write buffer="DE\nDR1\nCH1;CH2\nCH1, 'V1','I1',2,1\nCH2,'COM','GND',3,3\nSS\nIL1, 1, 20, -.001,.001\nDT 0\nIT2\nRS 5\nRG 1, 100e-9\nRG 2, 100e-9\nSM\nDM2\nLI 'V1', 'I1'\nSM\nDM1\nXN 'I1', 1, -1E-9, 1E-9\nYA 'V1', 1, -1E-7,1E-7\nMD\nME1\n", error in (no error)=w402) -> (VISA resource name out=w405:refnum<visa-resource-name>, error out=w406:errorcluster)  [unwired: 1 out]
        n224 = call <vilib>:"Wait for RQS.vi"("error in (no error)"=w406, "VISA resource name"=w405) -> ("error out"=w400:errorcluster, "VISA resource name out"=w401:refnum<visa-resource-name>)  [unwired: 1 in, 7 out]
        n225 = VISA Write(VISA resource name=w401, write buffer="DO 'I1'\n", error in (no error)=w400) -> (VISA resource name out=w452:refnum<visa-resource-name>, error out=w448:errorcluster)  [unwired: 1 out]
        n226 = VISA Read(VISA resource name=w452, byte count=u32 16000, error in (no error)=w448) -> (VISA resource name out=w450:refnum<visa-resource-name>, read buffer=w435:string, error out=w446:errorcluster)  [unwired: 1 out]
        n227 = Spreadsheet String To Array(delimiter (Tab)=",", format string="N %g", spreadsheet string=w435, array type (2D Dbl)=w442) -> (array=w439:dbl[])
        n228 = VISA Write(VISA resource name=w450, write buffer="DO 'V1'", error in (no error)=w446) -> (VISA resource name out=w444:refnum<visa-resource-name>, error out=w445:errorcluster)  [unwired: 1 out]
        n229 = VISA Read(VISA resource name=w444, byte count=u32 16000, error in (no error)=w445) -> (VISA resource name out=w454:refnum<visa-resource-name>, read buffer=w434:string, error out=w453:errorcluster)  [unwired: 1 out]
        n230 = Spreadsheet String To Array(delimiter (Tab)=",", format string="N %g", spreadsheet string=w434, array type (2D Dbl)=w442) -> (array=w438:dbl[])
        n231 = VISA Close(VISA resource name=w454, error in (no error)=w453) -> (error out=w394:errorcluster)
        n232 = Bundle(w439, w438) -> (→"XY Graph":cluster{dbl[], dbl[]})  [unwired: 1 in]
        n233 = Build Array(w439, w438) -> (w436:dbl[][])
        n234 = Transpose 2D Array(2D array=w436) -> (transposed array=w421:dbl[][])
        "Current (A)    Voltage (V)" <- w421
        n235 = Index Array(array=w421, index (row)=0, index (col)=0 ("index (row)")) -> (element=w424:dbl)
        n236 = Index Array(array=w421, index (row)=0, index (col)=1 ("index (row)")) -> (element=w422:dbl)
        n237 = Index Array(array=w421, index (row)=1, index (col)=0 ("index (row)")) -> (element=w425:dbl)
        n238 = Index Array(array=w421, index (row)=1, index (col)=1 ("index (row)")) -> (element=w423:dbl)
        n239 = Subtract(x=w423, y=w422) -> (x-y=w419:dbl)
        n240 = Subtract(x=w425, y=w424) -> (x-y=w420:dbl)
        n241 = Divide(x=w419, y=w420) -> (x/y=w393:dbl)
        "Resistance (Ohm)" <- w393
        n242 = Bundle(w393) -> (→"Waveform Chart 3":cluster{dbl})  [unwired: 1 in]
        n243 = Number To Engineering String(4:w393) -> (0:w395:string)  [unwired: 3 in]
      }
    }
    n244 = case shown="True" w363 {
      tunnel: [w483 w488] -> w385
      tunnel: w384 -> [w483 w497]
      tunnel: w382 -> [_ w489]
      tunnel: w379 -> [_ w490]
      tunnel: [w482 w484] -> w378
      frame False {
        w480 = "no GenAir data"
        n245 = Bundle("y"=0.0, w480, w480, "error out"=errorcluster {"status"=FALSE, "code"=0, "source"=""}) -> (w482:T11)  [unwired: 1 in]
      }
      frame True {
        # "SetNag O2 Gauge"
        # "SetNag O2 Pump Voltage"
        n246 = flat-sequence {
          tunnel: [w506] -> w503
          tunnel: w489 -> [w508]
          tunnel: w490 -> [w506]
          tunnel: w503 -> [w509]
          tunnel: w489 -> [w516]
          tunnel: [w512] -> w488
          frame #0 {
            n247 = Wait (ms)(milliseconds to wait=w508) -> ()  [unwired: 1 out]
            n248 = call <vilib>:"Serial Port Write.vi"("string to write"="_OXY\r" ("O2 partial press"), "port number"=w506) -> ()  [unwired: 1 out]
          }
          frame #1 {
            # "O2 partial pressure"
            n249 = call <vilib>:"Bytes At Serial Port.vi"() -> ("byte count"=w517:u32)  [unwired: 1 in, 1 out]
            n250 = Wait (ms)(milliseconds to wait=w516) -> ()  [unwired: 1 out]
            n251 = call <vilib>:"Serial Port Read.vi"("requested byte count"=w517, "port number"=w509) -> ("string read"=w515:string)  [unwired: 1 out]
            n252 = Fract/Exp String To Number(string=w515) -> (number=w513:dbl)  [unwired: 3 in, 1 out]
            "atm" <- w513
            n253 = Multiply(x=w513, y=100.0) -> (x*y=w510:dbl)
            "%" <- w510
            n254 = Multiply(x=w510, y=7.6) -> (x*y=w512:dbl)
            "Torr" <- w512
          }
        }
        n255 = call <vilib>:"DAQmx Start Task.vi"("task/channels in"=refnum<k21> "SetNag_Pump_Voltage") -> ("task out"=w492:refnum<k21>, "error out"=w491:errorcluster)  [unwired: 13 in]
        n256 = call-poly <vilib>:"DAQmx Read.vi"("task/channels in"=w492, "error in"=w491) -> ("task out"=w495:refnum<k21>, "data"=w496:dbl, "error out"=w494:errorcluster)  [unwired: 11 in]
        "Waveform Chart 2" <- w496
        "O2 pump voltage" <- w496
        n257 = call <vilib>:"DAQmx Stop Task.vi"("task/channels in"=w495, "error in"=w494) -> ("error out"=w485:errorcluster)  [unwired: 12 in, 1 out]
        n258 = Number To Engineering String(4:w496) -> (0:w486:string)  [unwired: 3 in]
        n259 = Greater?(x=w488, y=1e-07) -> (0:w499:bool)
        n260 = case shown="False" w499 {
          tunnel: [w504 w505] -> w498
          tunnel: w488 -> [_ w505]
          tunnel: w497 -> [w504 _]
          frame False {
          }
          frame True {
          }
        }
        n261 = Number To Engineering String(4:w498) -> (0:w487:string)  [unwired: 3 in]
        n262 = Bundle(w487) -> (w501:cluster{string})  [unwired: 1 in]
        n263 = Fract/Exp String To Number(string=w501) -> (number=→"Waveform Chart":cluster{dbl})  [unwired: 3 in, 1 out]
        n264 = Bundle(w488, w487, w486, "error out"=w485) -> (w484:T12)  [unwired: 1 in]
      }
    }
    n265 = Wait (ms)(milliseconds to wait=w382) -> ()  [unwired: 1 out]
    n266 = case shown="False" w368 {
      tunnel: w383 -> [_ w470]
      tunnel: [w457 w462] -> w377
      tunnel: w374 -> [_ w461]
      frame False {
        w455 = "no QCM data"
        n267 = Bundle("error out"=errorcluster {"status"=FALSE, "code"=0, "source"=""}, w455, w455) -> (w457:T13)  [unwired: 1 in]
      }
      frame True {
        w469 = 1000  # chart length (points)
        # "SRS QCM"
        n268 = Unbundle(w461) -> ("Elapsed Time (s)"=w460:dbl, "VISA out"=w459:refnum<visa-resource-name>, "error out"=w458:errorcluster)
        n269 = Equal To 0?(x=w470) -> (x = 0?=w473:bool)
        n270 = call <instrlib>:"SrsQcm200FandR.vi"("VISA in"=w459, "Reference time in"=w460, "error in (no error)"=w458) -> ("VISA out"=w467:refnum<visa-resource-name>, "Frequency out"=w472:dbl, "Resistance out"=w471:dbl, "F vs T out"=w478:T14, "R vs T out"=w477:T15, "error out"=w466:errorcluster)  [unwired: 6 in, 1 out]
        "Frequency (Hz)" <- w472
        "Resistance (Ohm)" <- w471
        n271 = call <instrlib>:"XY Chart Buffer.vi"("clear first (no:F)"=w473, "chart length (points)"=w469, "new point"=w478) -> ("XY chart data"=w475:cluster{"x":dbl, "y":dbl}[])  [unwired: 8 in]
        n272 = call <instrlib>:"XY Chart Buffer.vi"("clear first (no:F)"=w473, "chart length (points)"=w469, "new point"=w477) -> ("XY chart data"=w476:cluster{"x":dbl, "y":dbl}[])  [unwired: 8 in]
        n273 = call <instrlib>:"srsQcm200Close.vi"("error in"=w466, "Visa in"=w467) -> ("error out"=w468:errorcluster)  [unwired: 3 in]
        n274 = call <vilib>:"Simple Error Handler.vi"("error in (no error)"=w468) -> ("error out"=w465:errorcluster)  [unwired: 4 in, 4 out]
        n275 = Build Cluster Array(w476, w475) -> (→"Freq and Resistance Graph 2":T2)
        n276 = Number To Engineering String(4:w471) -> (0:w463:string)  [unwired: 3 in]
        n277 = Number To Engineering String(4:w472) -> (0:w464:string)  [unwired: 3 in]
        n278 = Bundle("error out"=w465, w464, w463) -> (w462:T13)  [unwired: 1 in]
      }
    }
    n279 = Unbundle(w377) -> ("error out"=w371:errorcluster, w376:string, w375:string)
    n280 = Unbundle(w378) -> (w373:string, w372:string, "error out"=w369:errorcluster)  [unwired: 1 out]
    n281 = Get Date/Time In Seconds() -> (seconds since 1Jan1904=w389:timestamp)
    n282 = call "Elapsed Time"() -> ("Elapsed Time (s)"=w381:dbl)  [unwired: 12 in, 7 out]
    n283 = Format Date/Time String(seconds (now)=w389) -> (date/time string=w386:string)  [unwired: 2 in]
    "Current Date/Time" <- w386
    n284 = Number To Engineering String(4:w381) -> (0:w387:string)  [unwired: 3 in]
    n285 = Bundle("error out"=w371, "error out"=w369, "error out"=w361) -> (w370:T16)  [unwired: 1 in]
    n286 = Build Array(w386, w387, w376, w375, w373, w372, w362, "Add comments to the data file here and click anywhere outside the comment\nbox to save. The time at which the comment is saved is recorded in the data file.") -> (w367:string[])
  }
  n287 = Unbundle(w16) -> ("error out"=w15:errorcluster, "error out"=w14:errorcluster, "error out"=w1:errorcluster)
  n288 = Merge Errors(w15, w14, w1, w6) -> (w13:errorcluster)
  n289 = call <vilib>:"Simple Error Handler.vi"("error in (no error)"=w13) -> ("error out"=→"Program Errors":errorcluster)  [unwired: 4 in, 4 out]
  n290 = Not(x=w3) -> (.not. x?=w2:bool)
  n291 = case shown="True" w3 {
    tunnel: w11 -> [_ w520]
    frame False {
    }
    frame True {
      n292 = call <instrlib>:"OpenCreateReplace File.vi"("prompt"="Choose the file path for the  instrument data", "function (open:0)"=T3."create or replace") -> ("new file path"=w519:path)  [unwired: 6 in, 3 out]
      n293 = Build Array("date/time", "elapsed time (s)", "QCM freq (Hz)", "QCM resistance (Ohm)", "O2 partial pressure (Torr)" ("element"), "O2 pump voltage (V)" ("element"), "Keithley 4-point resistance (Ohm) " ("element"), "user comment" ("element")) -> (w524:string[])
      n294 = call-poly <vilib>:"Write To Spreadsheet File.vi"("1D data"=w524, "file path (dialog if empty)"=w519) -> ("new file path (Not A Path if cancelled)"=w525:path)  [unwired: 6 in]
      n295 = call-poly <vilib>:"Write To Spreadsheet File.vi"("append to file? (new file:F)"=TRUE, "2D data"=w520, "file path (dialog if empty)"=w525) -> ()  [unwired: 5 in, 1 out]
    }
  }
  n296 = call "Display Message to User"("Enable"=w2) -> ()  [unwired: 9 in, 2 out]
